vi "Write Gantry Head.vi"(8 "error in":errorcluster, 10 "Gantry Head":T1, 11 "WorkTable in":refnum<class "WorkTable Class.lvclass">) -> (0 "error out":errorcluster, 3 "WorkTable out":refnum<class "WorkTable Class.lvclass">)   [LabVIEW 2011, in "WorkTable Class.lvclass"]
uses:
  WorkTable Class.lvclass
  Type Definitions/Worktable_Gantry Head.ctl
  WorkTable Class.lvclass/WorkTable Class.ctl
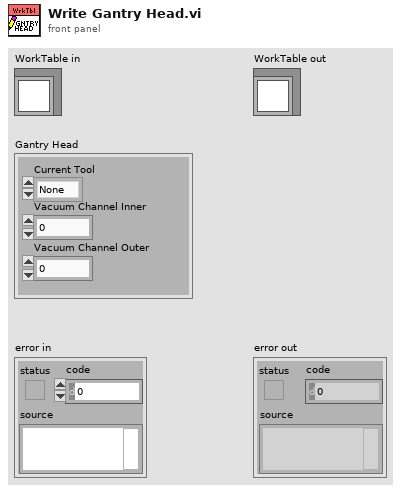
[diagram p1: front panel]
types:
  T1 = typedef "Worktable_Gantry Head.ctl" = cluster{"Current Tool":enum16{"None", "Grabber", "Picker", "Tool Setter"}, "Vacuum Channel Inner":i32, "Vacuum Channel Outer":i32}
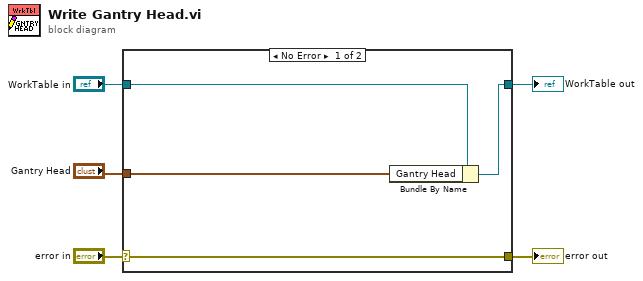
[diagram p0: block diagram]
diagram:
  n1 = case shown="No Error" "error in" {
    selector: "error in" -> [w9 w10]
    tunnel: [w9 w10] -> w4
    tunnel: [w7 w11] -> w2
    tunnel: "WorkTable in" -> [w8 w11]
    tunnel: "Gantry Head" -> [w6 _]
    frame No Error {
      n2 = Bundle By Name(cluster=w8, "Gantry Head"=w6) -> (w7:refnum<class "WorkTable Class.lvclass">)
    }
    frame Error {
    }
  }
  "error out" <- w4
  "WorkTable out" <- w2
